vi "Toggle Debug Visible.vi"(8 "error in (no error)":errorcluster, 10 "Visible":bool, 11 "Rename in":refnum<class "Rename.lvclass">) -> (0 "error out":errorcluster, 3 "Rename out":refnum<class "Rename.lvclass">)   [LabVIEW 2015, in "Generic Module Library.lvlib" / "Template G_Module.lvlib" / "Rename.lvclass"]
uses:
  Rename.lvclass
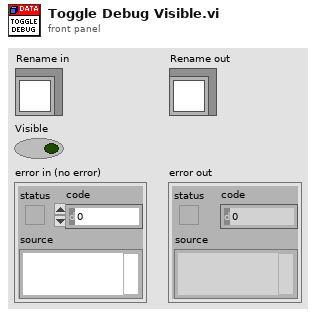
[diagram p1: front panel]
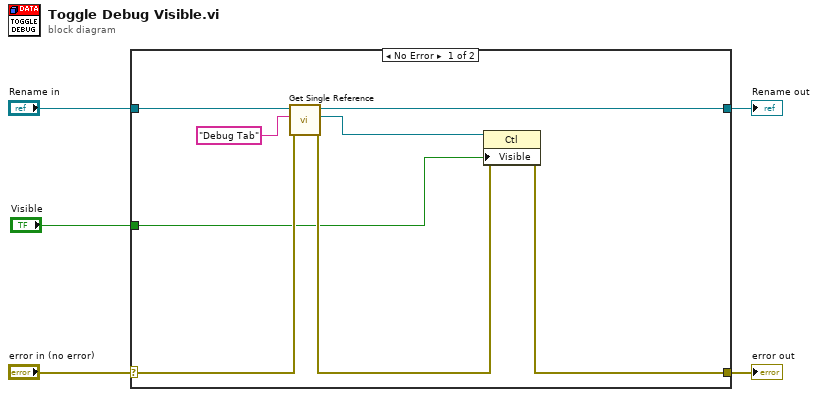
[diagram p0: block diagram]
diagram:
  n1 = case shown="No Error" "error in (no error)" {
    selector: "error in (no error)" -> [w11 w15]
    tunnel: [w7 w15] -> w4
    tunnel: [w12 w14] -> w2
    tunnel: "Rename in" -> [w13 w14]
    tunnel: "Visible" -> [w6 _]
    frame No Error {
      n2 = call "Get Single Reference.vi"("error in (no error)"=w11, "Control Name"="Debug Tab", "Rename in"=w13) -> ("error out"=w8:errorcluster, "Control Reference"=w9:refnum<vi>, "Rename out"=w12:refnum<class "Rename.lvclass">)  [unwired: 6 in]
      n3 = property class="Ctl"(reference=w9, error in=w8, "Visible"=w6) -> (error out=w7:errorcluster)  [unwired: 1 out]
    }
    frame Error {
    }
  }
  "error out" <- w4
  "Rename out" <- w2
